vi "BarcodeSN Input.vi"(10 "位數":i32=9, 11 "String Input":string="0872j12701.A46007") -> (3 "Array":u16[](array[numeric]))   [LabVIEW 2019]
panel:
  out "(hi.lo) 7":u16
  out "element 12":u8
  out "element 11":u8
  out "(hi.lo) 6":u16
  out "element 10":u8
  out "element 9":u8
  out "(hi.lo) 5":u16
  out "element 8":u8
  out "element 7":u8
  out "(hi.lo) 4":u16
  out "element 6":u8
  out "element 5":u8
  out "(hi.lo) 3":u16
  out "element 4":u8
  out "element 3":u8
  out "(hi.lo) 2":u16
  out "String":string
  out "unsigned byte array":u8[](array[numeric])
  out "element":u8
  out "element 2":u8
  out "(hi.lo)":u16
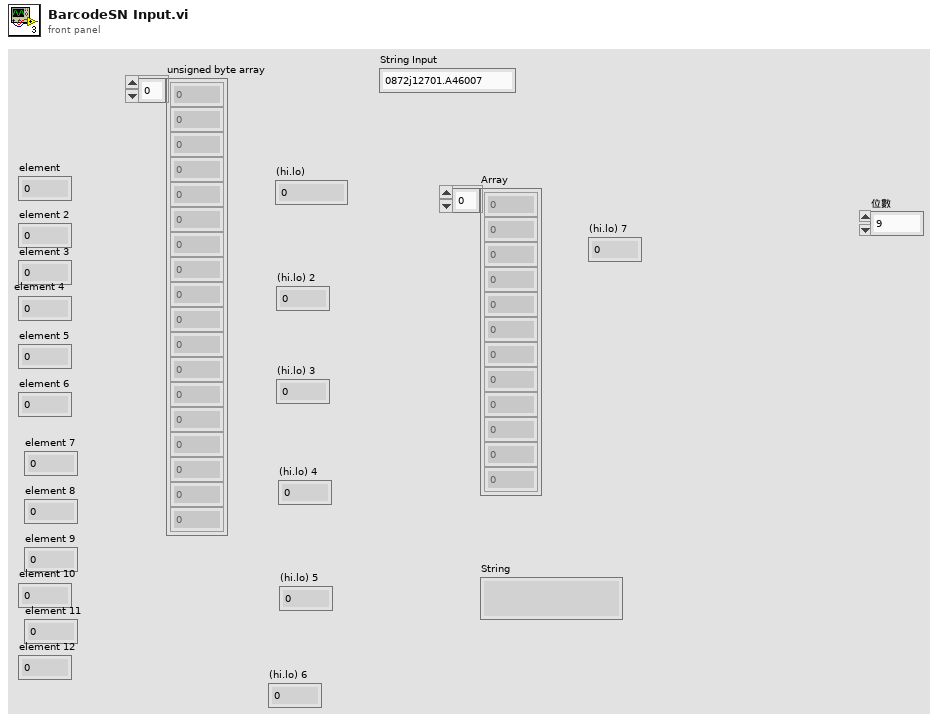
[diagram p1: front panel]
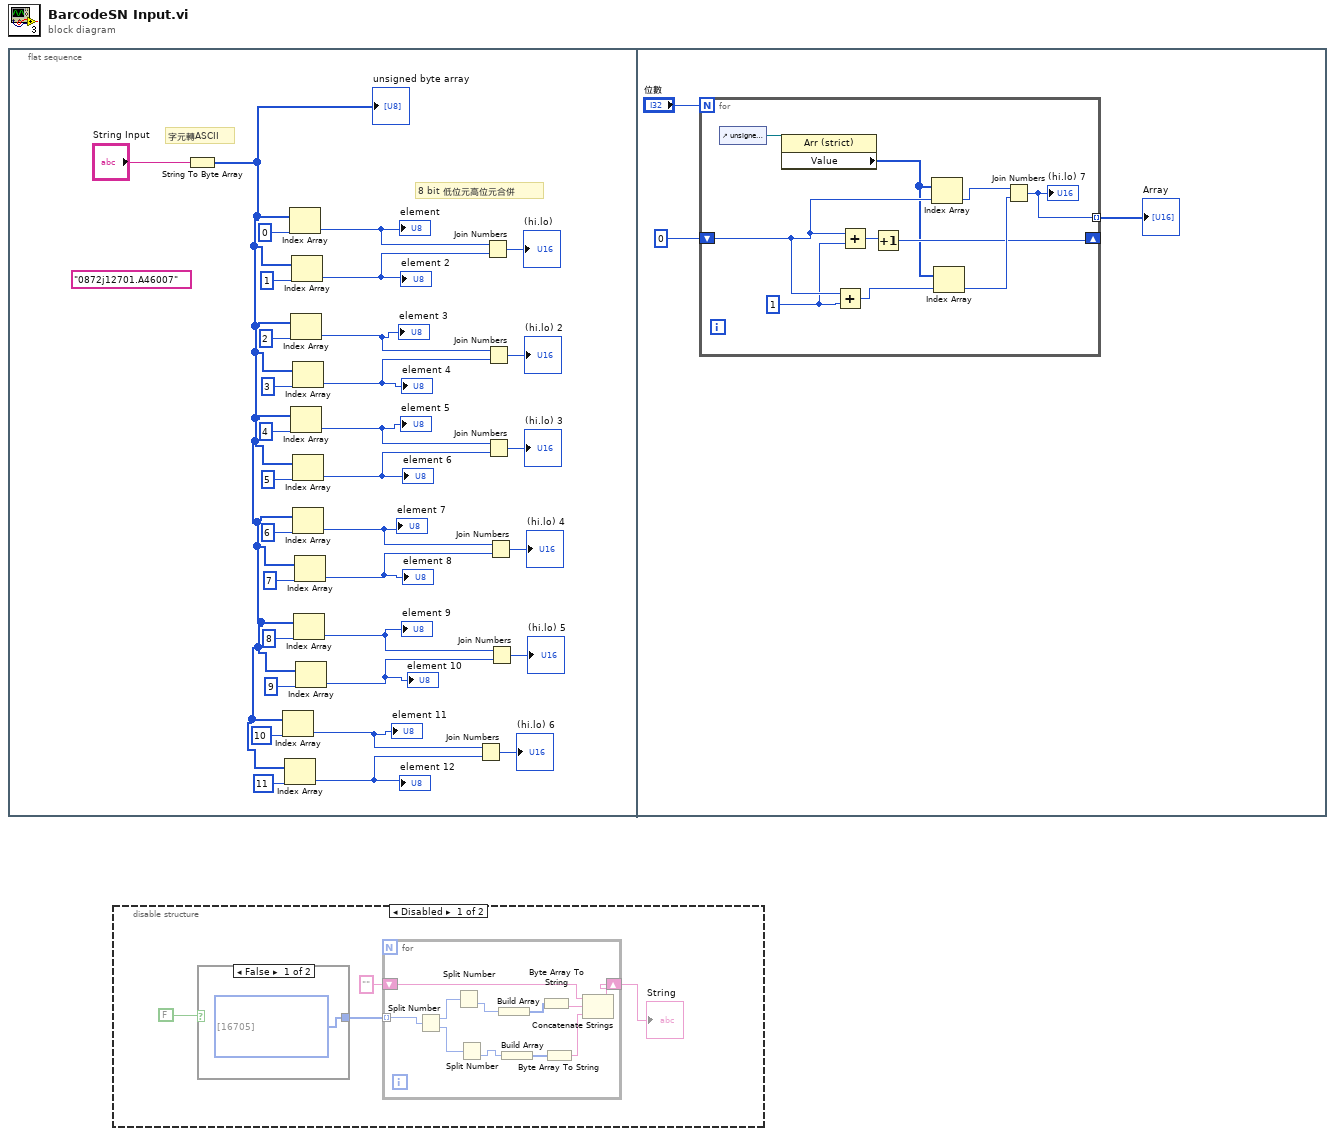
[diagram p0: block diagram]
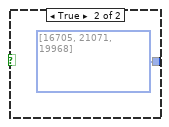
[diagram p2: hidden frame]
diagram:
  n1 = flat-sequence {
    frame #0 {
      (unwired) "0872j12701.A46007"
      # "8 bit 低位元高位元合併"
      # "字元轉ASCII"
      n2 = String To Byte Array(string="String Input") -> (unsigned byte array=w12:u8[])
      "unsigned byte array" <- w12
      n3 = Index Array(array=w12, index=10) -> (element=w3:u8)
      "element 11" <- w3
      n4 = Index Array(array=w12, index=11) -> (element=w2:u8)
      "element 12" <- w2
      n5 = Index Array(array=w12, index=0) -> (element=w30:u8)
      "element" <- w30
      n6 = Index Array(array=w12, index=2) -> (element=w11:u8)
      "element 3" <- w11
      n7 = Index Array(array=w12, index=4) -> (element=w9:u8)
      "element 5" <- w9
      n8 = Index Array(array=w12, index=1) -> (element=w31:u8)
      "element 2" <- w31
      n9 = Index Array(array=w12, index=3) -> (element=w10:u8)
      "element 4" <- w10
      n10 = Index Array(array=w12, index=5) -> (element=w8:u8)
      "element 6" <- w8
      n11 = Index Array(array=w12, index=6) -> (element=w7:u8)
      "element 7" <- w7
      n12 = Index Array(array=w12, index=8) -> (element=w5:u8)
      "element 9" <- w5
      n13 = Index Array(array=w12, index=7) -> (element=w6:u8)
      "element 8" <- w6
      n14 = Index Array(array=w12, index=9) -> (element=w4:u8)
      "element 10" <- w4
      n15 = Join Numbers(hi=w3, lo=w2) -> ((hi.lo)=→"(hi.lo) 6":u16)
      n16 = Join Numbers(hi=w30, lo=w31) -> ((hi.lo)=→"(hi.lo)":u16)
      n17 = Join Numbers(hi=w11, lo=w10) -> ((hi.lo)=→"(hi.lo) 2":u16)
      n18 = Join Numbers(hi=w9, lo=w8) -> ((hi.lo)=→"(hi.lo) 3":u16)
      n19 = Join Numbers(hi=w7, lo=w6) -> ((hi.lo)=→"(hi.lo) 4":u16)
      n20 = Join Numbers(hi=w5, lo=w4) -> ((hi.lo)=→"(hi.lo) 5":u16)
    }
    frame #1 {
      n21 = for {
        N: "位數" -> [_]
        shift-right: [w40] -> _
        shift-left: 0 -> [w42]
        tunnel: [w38] -> w34 mode=indexing
        w39 = 1
        n22 = control-ref of="unsigned byte array"() -> (w37:refnum<vi>)
        n23 = property class="Arr (strict)"(reference=w37) -> ("Value"=w36:u8[])  [unwired: 1 in, 2 out]
        n24 = Add(x=w42, y=w39) -> (x+y=w43:i32)
        n25 = Add(x=w42, y=w39) -> (x+y=w41:i32)
        n26 = Increment(x=w41) -> (x+1=w40:i32)
        n27 = Index Array(array=w36, index=w42) -> (element=w45:u8)
        n28 = Index Array(array=w36, index=w43) -> (element=w44:u8)
        n29 = Join Numbers(hi=w45, lo=w44) -> ((hi.lo)=w38:u16)
        "(hi.lo) 7" <- w38
      }
      "Array" <- w34
    }
  }
  n30 = disable-structure shown="Disabled" {
    frame Disabled {
      n31 = case shown="False" FALSE {
        tunnel: [u16[] [16705] ("unsigned byte array") u16[] [16705, 21071, 19968] ("unsigned byte array")] -> w46
        frame False {
        }
        frame True {
        }
      }
      n32 = for {
        tunnel: w46 -> [w62] mode=indexing
        shift-right: [w54] -> w48
        shift-left: "" -> [w55]
        n33 = Split Number(x=w62) -> (hi(x)=w60:u8, lo(x)=w58:u8)
        n34 = Split Number(x=w60) -> (lo(x)=w53:u8)  [unwired: 1 out]
        n35 = Split Number(x=w58) -> (lo(x)=w52:u8)  [unwired: 1 out]
        n36 = Build Array(w53) -> (w61:u8[])
        n37 = Build Array(w52) -> (w59:u8[])
        n38 = Byte Array To String(unsigned byte array=w61) -> (string=w57:string)
        n39 = Byte Array To String(unsigned byte array=w59) -> (string=w56:string)
        n40 = Concatenate Strings(w55, w57, w56) -> (w54:string)
      }
      "String" <- w48
    }
    frame Enabled {
    }
  }
